vi "U16 to Hex.vi"(11 "number":dbl) -> (3 "Hex string":string)   [LabVIEW 2013]
panel:
  out "hex integer string":string
  # "RE-ENTRANT"
  # "SUBROUTINE"
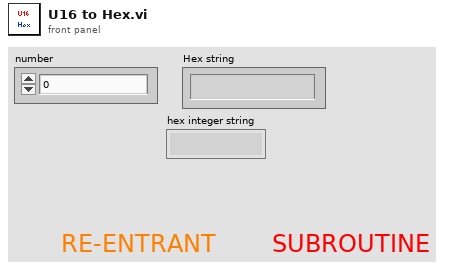
[diagram p1: front panel]
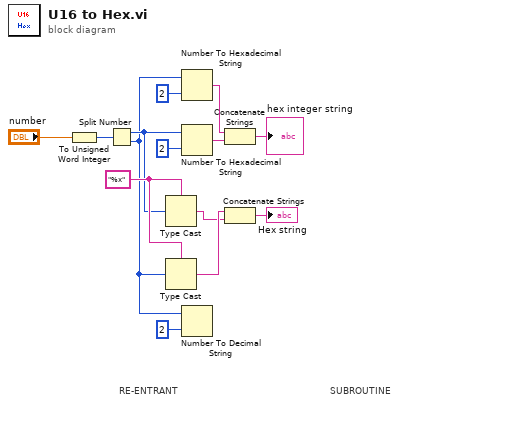
[diagram p0: block diagram]
diagram:
  w7 = "%x" ("type")
  # "SUBROUTINE"
  # "RE-ENTRANT"
  n1 = To Unsigned Word Integer(number="number") -> (unsigned 16bit integer=w12:u16)
  n2 = Split Number(x=w12) -> (hi(x)=w4:u8, lo(x)=w3:u8)
  n3 = Type Cast(type=w7, x=w4) -> (*(type *) &x=w1:string)
  n4 = Type Cast(type=w7, x=w3) -> (*(type *) &x=w2:string)
  n5 = Number To Hexadecimal String(1:i16 2 ("width (-)"), 2:w3) -> (0:w14:string)
  n6 = Number To Hexadecimal String(1:i16 2 ("width (-)"), 2:w4) -> (0:w13:string)
  n7 = Number To Decimal String(number=w3, width (-)=i16 2) -> ()  [unwired: 1 out]
  n8 = Concatenate Strings(w14, w13) -> (→"hex integer string":string)
  n9 = Concatenate Strings(w2, w1) -> (→"Hex string":string)
